vi "Logging Active.vi"(8 "error in (no error)":errorcluster, 10 "Context in":refnum<class "Context.lvclass">, 11 "Active in":refnum<class "Active.lvclass">) -> (0 "error out":errorcluster, 2 "Context out":refnum<class "Context.lvclass">, 3 "State out":refnum<class "State.lvclass">)   [LabVIEW 2024, in "State.lvlib" / "Active.lvclass"]
uses:
  Active.lvclass
  Active.lvclass/Active.ctl
  Logging/Logging.lvclass
  State/State.lvclass
  C:/Users/uspoaotto/OneDrive - Oregon Tool/Desktop/working copies/stateMachineActor/src/State Machine/State/State/State.lvclass
  C:/Users/uspoaotto/OneDrive - Oregon Tool/Desktop/working copies/stateMachineActor/src/State Machine/State/~State/~State.lvclass
  C:/Users/uspoaotto/OneDrive - Oregon Tool/Desktop/working copies/stateMachineActor/src/State Machine/State/Active/Active.lvclass
  C:/Users/uspoaotto/OneDrive - Oregon Tool/Desktop/working copies/stateMachineActor/src/State Machine/State/Logging/Logging.lvclass
  Context/Context/Context.lvclass
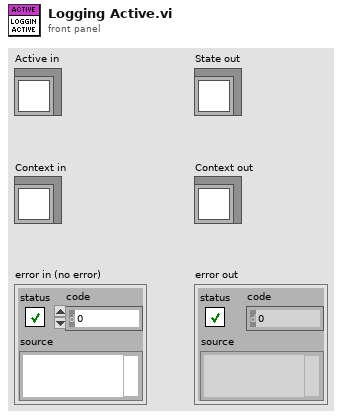
[diagram p1: front panel]
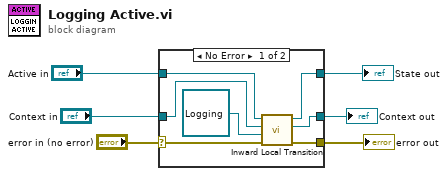
[diagram p0: block diagram]
diagram:
  n1 = case shown="No Error" "error in (no error)" {
    selector: "error in (no error)" -> [w10 w15]
    tunnel: "Active in" -> [w12 w16]
    tunnel: [w8 w16] -> w5
    tunnel: [w9 w15] -> w4
    tunnel: "Context in" -> [w13 w14]
    tunnel: [w7 w14] -> w1
    frame No Error {
      n2 = call "Inward Local Transition.vi"("error in (no error)"=w10, "Target State"=refnum<class "Logging.lvclass"> refnum ("State.lvlib:Logging.lvclass"), "Context in"=w13, "State in"=w12) -> ("error out"=w9:errorcluster, "Context out"=w7:refnum<class "Context.lvclass">, "State out"=w8:refnum<class "State.lvclass">)  [unwired: 5 in]
    }
    frame Error {
    }
  }
  "error out" <- w4
  "State out" <- w5
  "Context out" <- w1
